vi "YawZeroGlobal.vi"(11 "Update":bool) -> (3 "YawZero":dbl)   [LabVIEW 2014, in "Nav6.lvlib"]
uses:
  Nav6.lvlib
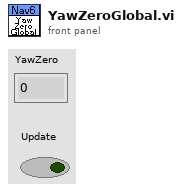
[diagram p1: front panel]
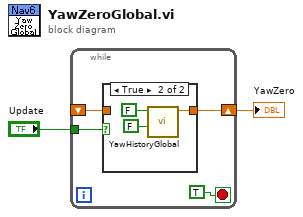
[diagram p0: block diagram]
diagram:
  n1 = while {
    tunnel: "Update" -> [w6]
    shift-right: [w4] -> w1
    shift-left: _ -> [w3]
    stop <- TRUE stop-if-true
    n2 = case shown="True" w6 {
      tunnel: [w7 w9] -> w4
      tunnel: w3 -> [w7 _]
      frame False {
      }
      frame True {
        n3 = call "YawHistoryGlobal.vi"("Initialize"=FALSE, "Update"=FALSE) -> ("Average Yaw History"=w9:dbl)  [unwired: 9 in]
      }
    }
  }
  "YawZero" <- w1
